vi "GetType.vi"(8 "error in (no error)":errorcluster, 11 "Abort Msg":refnum<class "Abort Msg.lvclass">) -> (0 "error out":errorcluster, 2 "Data Sample":variant, 3 "Abort Msg":refnum<class "Abort Msg.lvclass">)   [LabVIEW 2015, in "CS++Scope.lvlib" / "Abort Msg.lvclass"]
doc: "This VI delivers a sample of the data type format the message expects."
uses:
  Abort Msg.lvclass
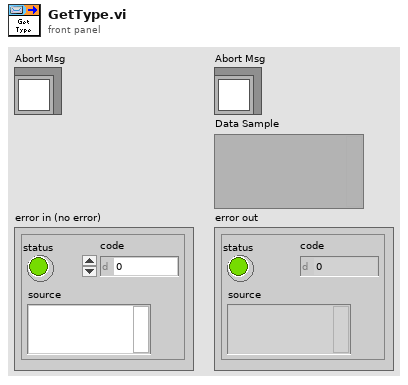
[diagram p1: front panel]
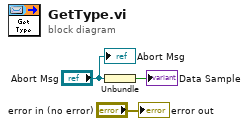
[diagram p0: block diagram]
diagram:
  n1 = Unbundle("Abort Msg") -> (→"Data Sample":bool)
  "error out" <- "error in (no error)"
  "Abort Msg" <- "Abort Msg"
